vi "IDE_Folder_Example.vi"() -> ()   [LabVIEW 2020]
uses:
  Subs/ColorText/Code.xctl
  Subs/Console XCtrl/Console_Xctrl.xctl
  Subs/Server XCtrl/Server.xctl
panel:
  in  "Base Path":path
  in  "Tree":string(tree)
  in  "Clean":bool
  in  "PC Save":bool
  in  "Files":bool
  in  "Server":bool
  in  "Help":bool
  in  "Server":path(xcontrol)=path "/Users/crogers/GitHub/Summer2020/LabVIEWCode/Servers/Jens.vi"
  out "REPL":string(xcontrol)
  in  "Clear":bool
  in  "Save":bool
  in  "Stop":bool
  in  "Run":bool
  in  "Name":string="code.py"
  in  "Code":string(xcontrol)="import os\n\nfor i in range(10):\n     print(i)\n"
  # "¨Processor"
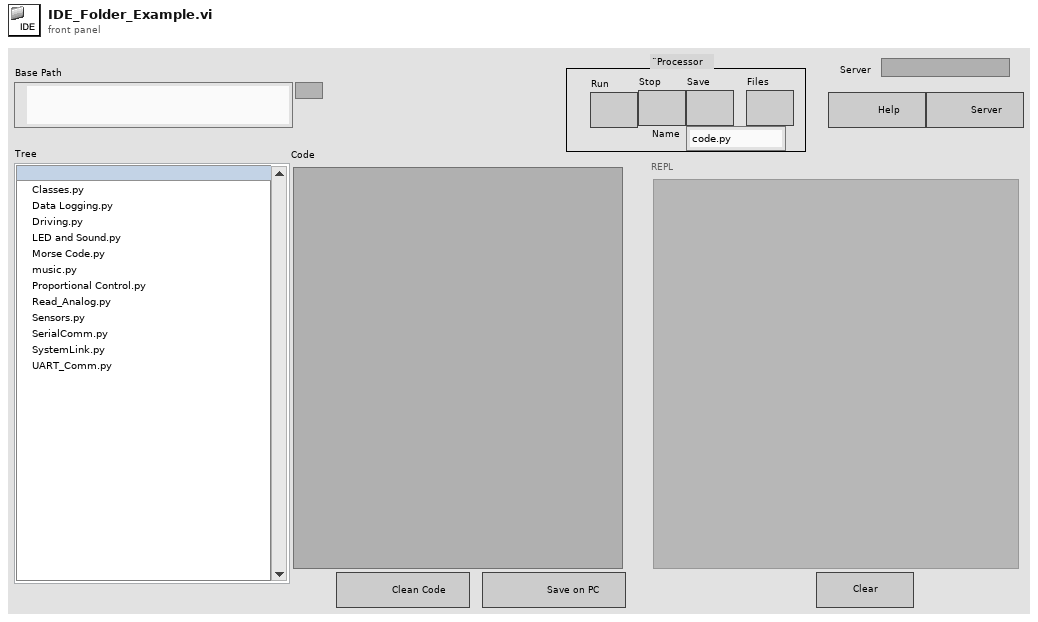
[diagram p1: front panel]
types:
  T1 = cluster{"Quote":u32, "Comment":u32, "Python":u32, "Text":u32, "Triple Quote":u32, "function":u32, "Line numbers":u32, "REPL Err":u32, "REPL Text":u32, "Text Bkgd":u32, "REPL Bkgd":u32}
  T2 = enum8{"Enabled", "Disabled", "Disabled and Grayed Out"}
  T3 = typedef "eventvkey.ctl" = enum16{"ASCII", "Enter", "Return", "Shift", "Ctrl", "Alt", "Cmd", "Opt", "Caps", "NumLock", "Clear", "Break", "Up", "Down", "Left", "Right", "Insert", "Delete", "Home", "End", "PageUp", "PageDown", "Escape", "Help", "Pause", "ScrollLock", "F1", "F2", "F3", "F4", "F5", "F6", "F7", "F8", "F9", "F10", "F11", "F12", "F13", "F14", "F15", "F16", "F17", "F18", "F19", "F20", "F21", "F22", "F23", "F24", "Play", "VolumeUp", "VolumeDown", "Mute", "Two Byte Char"}
  T4 = cluster{"Shift":bool, "Ctrl":bool, "Alt":bool, "Cmd":bool, "Opt":bool}
  T5 = cluster{"Char":i16, "VKey":T3, "PlatMods":cluster{"Shift":bool, "Ctrl":bool, "Alt":bool, "Cmd":bool, "Opt":bool}}
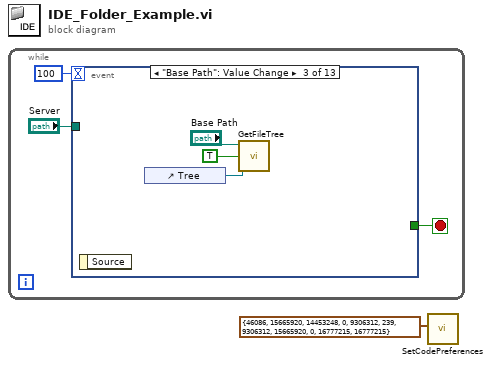
[diagram p0: block diagram]
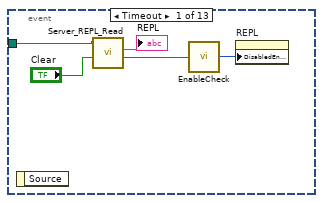
[diagram p2: hidden frame]
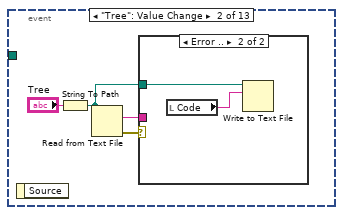
[diagram p3: hidden frame]
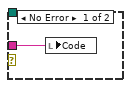
[diagram p4: hidden frame]
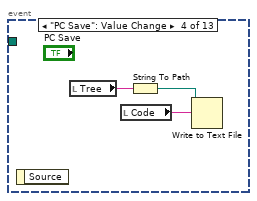
[diagram p5: hidden frame]
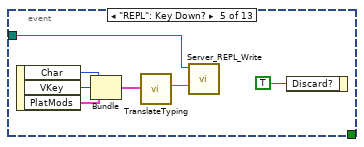
[diagram p6: hidden frame]
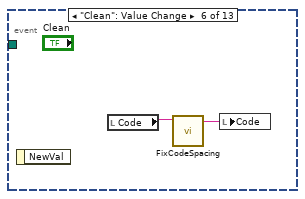
[diagram p7: hidden frame]
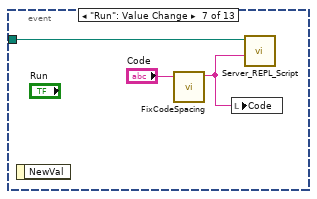
[diagram p8: hidden frame]
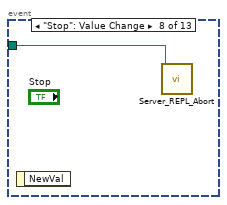
[diagram p9: hidden frame]
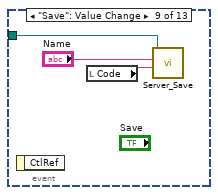
[diagram p10: hidden frame]
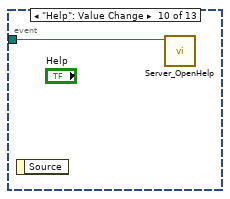
[diagram p11: hidden frame]
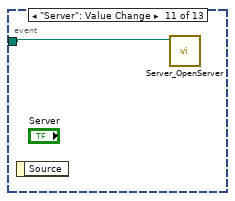
[diagram p12: hidden frame]
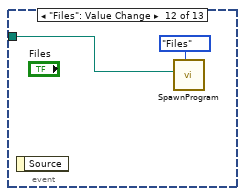
[diagram p13: hidden frame]
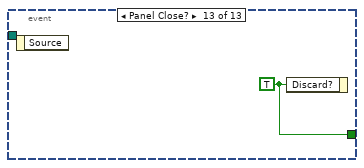
[diagram p14: hidden frame]
diagram:
  n1 = while {
    stop <- w3 stop-if-true
    n2 = event shown="[2] \"Base Path\": Value Change" {
      selector: _ -> [_ _ _ _ _ _ _ _ _ _ _ _ _]
      dyn-events: _ -> [_ _ _ _ _ _ _ _ _ _ _ _ _]
      timeout: 100 -> [_ _ _ _ _ _ _ _ _ _ _ _ _]
      tunnel: [_ _ _ _ _ _ _ _ _ _ _ _ w43] -> w3
      tunnel: "Server" -> [w7 _ _ _ w23 _ w33 w35 w36 w39 w40 w42 _]
      event Timeout {
        n3 = event-data() -> ()  [unwired: 1 in, 1 out]
        n4 = call "Server_REPL_Read.vi"("Clear"="Clear", "Server"=w7) -> ("Running?"=w8:bool, "REPL"=→"REPL":string)  [unwired: 7 in, 1 out]
        n5 = call "EnableCheck.vi"("Enable?"=w8) -> ("Enum"=w9:T2)
        n6 = property on="REPL" class="Console_Xctrl (strict)"("DisabledEnum"=w9) -> ()  [unwired: 2 in, 2 out]
      }
      event "Tree": Value Change {
        n7 = event-data() -> ()  [unwired: 1 in, 1 out]
        n8 = String To Path(string="Tree") -> (path=w10:path)
        n9 = Read from Text File(file (use dialog)=w10) -> (text=w12:string, error out=w13:errorcluster)  [unwired: 3 in, 2 out]
        n10 = case shown="Error .." w13 {
          tunnel: w12 -> [w14 _]
          tunnel: w10 -> [_ w16]
          frame No Error {
            n11 = local write "Code"(w14) -> ()
          }
          frame Error {
            n12 = local read "Code"() -> (w15:string)
            n13 = Write to Text File(file (use dialog)=w16, text=w15) -> ()  [unwired: 2 in, 3 out]
          }
        }
      }
      event "Base Path": Value Change {
        n14 = event-data() -> ()  [unwired: 1 in, 1 out]
        n15 = control-ref of="Tree"() -> (w19:refnum<vi>)
        n16 = call "GetFileTree.vi"("Tree"=w19, "Open?"=TRUE, "Base Path"="Base Path") -> ()  [unwired: 9 in]
      }
      event "PC Save": Value Change {
        n17 = event-data() -> ()  [unwired: 1 in, 1 out]
        n18 = local read "Tree"() -> (w21:string)
        n19 = local read "Code"() -> (w22:string)
        n20 = String To Path(string=w21) -> (path=w20:path)
        n21 = Write to Text File(file (use dialog)=w20, text=w22) -> ()  [unwired: 2 in, 3 out]
      }
      event "REPL": Key Down? {
        n22 = event-data() -> ("Char"=w28:i16, "VKey"=w27:T3, "PlatMods"=w25:T4)  [unwired: 1 in]
        n23 = Bundle("Char"=w28, "VKey"=w27, "PlatMods"=w25) -> (w29:T5)  [unwired: 1 in]
        n24 = call "TranslateTyping.vi"("Cluster"=w29) -> ("key"=w24:string)  [unwired: 10 in]
        n25 = call "Server_REPL_Write.vi"("Code"=w24, "Server"=w23) -> ()  [unwired: 9 in, 1 out]
        n26 = event-data("Discard?"=TRUE) -> ()  [unwired: 1 in, 1 out]
      }
      event "Clean": Value Change {
        n27 = event-data() -> ()  [unwired: 1 in, 1 out]
        n28 = local read "Code"() -> (w30:string)
        n29 = call "FixCodeSpacing.vi"("Code"=w30) -> ("Cleaned"=w31:string)  [unwired: 10 in]
        n30 = local write "Code"(w31) -> ()
      }
      event "Run": Value Change {
        n31 = event-data() -> ()  [unwired: 1 in, 1 out]
        n32 = call "FixCodeSpacing.vi"("Code"="Code") -> ("Cleaned"=w32:string)  [unwired: 10 in]
        n33 = local write "Code"(w32) -> ()
        n34 = call "Server_REPL_Script.vi"("Code"=w32, "Server"=w33) -> ()  [unwired: 9 in, 1 out]
      }
      event "Stop": Value Change {
        n35 = event-data() -> ()  [unwired: 1 in, 1 out]
        n36 = call "Server_REPL_Abort.vi"("Server"=w35) -> ()  [unwired: 10 in, 1 out]
      }
      event "Save": Value Change {
        n37 = event-data() -> ()  [unwired: 1 in, 1 out]
        n38 = local read "Code"() -> (w38:string)
        n39 = call "Server_Save.vi"("Code"=w38, "Name"="Name", "Server"=w36) -> ()  [unwired: 8 in, 1 out]
      }
      event "Help": Value Change {
        n40 = event-data() -> ()  [unwired: 1 in, 1 out]
        n41 = call "Server_OpenHelp.vi"("Server"=w39) -> ()  [unwired: 10 in, 1 out]
      }
      event "Server": Value Change {
        n42 = event-data() -> ()  [unwired: 1 in, 1 out]
        n43 = call "Server_OpenServer.vi"("Server"=w40) -> ()  [unwired: 10 in, 1 out]
      }
      event "Files": Value Change {
        n44 = event-data() -> ()  [unwired: 1 in, 1 out]
        n45 = call "SpawnProgram.vi"("Server"=w42, "Dialog"=enum16{"Help", "Files"}."Files") -> ()  [unwired: 10 in]
      }
      event Panel Close? {
        w43 = TRUE ("Discard?")
        n46 = event-data() -> ()  [unwired: 1 in, 1 out]
        n47 = event-data("Discard?"=w43) -> ()  [unwired: 1 in, 1 out]
      }
    }
  }
  n48 = call "SetCodePreferences.vi"("Color choices"=T1 {"Quote"=46086, "Comment"=15665920, "Python"=14453248, "Text"=0, "Triple Quote"=9306312, "function"=239, "Line numbers"=9306312, "REPL Err"=15665920, "REPL Text"=0, "Text Bkgd"=16777215, "REPL Bkgd"=16777215}) -> ()  [unwired: 11 in]
